vi "adjust.vi"(8 "error in (no error)":errorcluster, 11 "DL090216RangeOffsetImageProcessor in":refnum<class "ImageProcessorDL090216RangeOffset.lvclass">) -> (0 "error out":errorcluster, 3 "DL090216RangeOffsetImageProcessor out":refnum<class "ImageProcessorDL090216RangeOffset.lvclass">)   [LabVIEW 2010, in "ImageProcessorDL090216RangeOffset.lvclass"]
uses:
  ImageProcessorDL090216RangeOffset.lvclass
  common/clusters/range_offset_cluster.ctl
  ImageProcessorDL090216RangeOffset.lvclass/ImageProcessorDL090216RangeOffset.ctl
  GenericImageProcessor/GenericImageProcessor/GenericImageProcessor.lvclass
  Command/GenericImageProcessorChangedCommand/GenericImageProcessorChangedCommand/GenericImageProcessorChangedCommand.lvclass
panel:
  in  "done":bool
  in  "channels":T1[](array[typedef]) {"offset" min=0.0 max=1.0 step=0.0010000000474974513 scale=0.0..1.0; "range" min=0.0 max=1.0 step=0.0010000000474974513 scale=0.0..1.0}
  in  "optimise":bool
  in  "master":T1={"range"=7.119999645510688e-05, "offset"=0.10570889711380005} {"offset" min=0.0 max=1.0 step=0.0010000000474974513 scale=0.0..1.0; "range" min=0.0 max=1.0 step=0.0010000000474974513 scale=0.0..1.0}
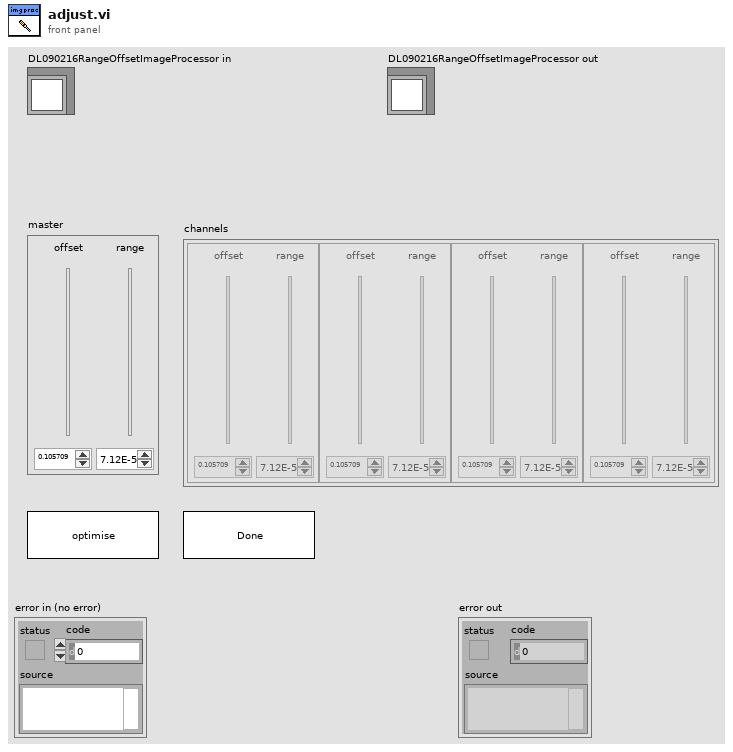
[diagram p1: front panel]
types:
  T1 = typedef "range_offset_cluster.ctl" = cluster{"range":dbl, "offset":dbl}
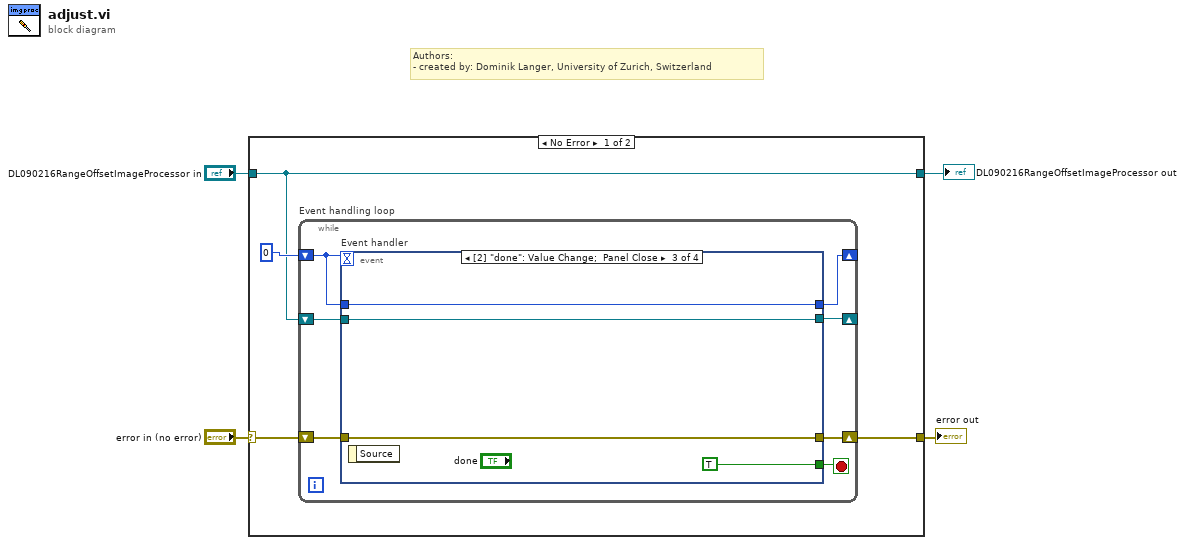
[diagram p0: block diagram]
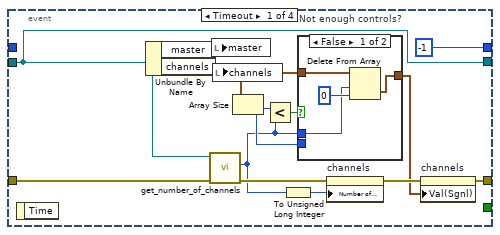
[diagram p2: hidden frame]
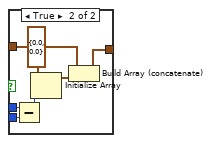
[diagram p3: hidden frame]
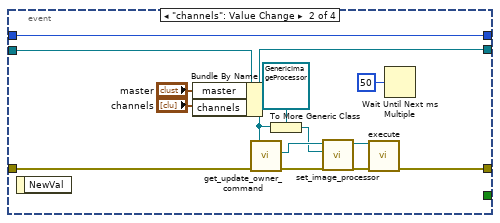
[diagram p4: hidden frame]
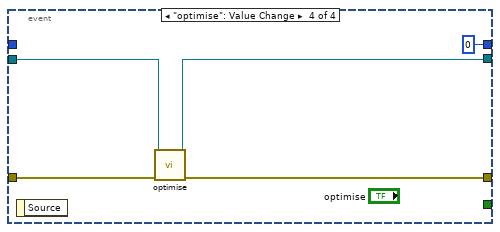
[diagram p5: hidden frame]
diagram:
  # "Authors: \n- created by: Dominik Langer, University of Zurich, Switzerland"
  n1 = case shown="No Error" "error in (no error)" {
    selector: "error in (no error)" -> [w8 w64]
    tunnel: [w7 w64] -> w3
    tunnel: [w5 w63] -> w2
    tunnel: "DL090216RangeOffsetImageProcessor in" -> [w5 w63]
    frame No Error {
      n2 = while "Event handling loop" {
        shift-right: [w14] -> w7
        shift-left: w8 -> [w15]
        shift-right: [w11] -> _
        shift-left: 0 -> [w12]
        shift-right: [w9] -> _
        shift-left: w5 -> [w10]
        stop <- w13 stop-if-true
        n3 = event "Event handler" shown="[2] \"done\": Value Change;  Panel Close" {
          selector: _ -> [_ _ _ _]
          dyn-events: _ -> [_ _ _ _]
          timeout: w12 -> [_ _ _ _]
          tunnel: w15 -> [w17 w49 w57 w59]
          tunnel: [w19 w51 w57 w58] -> w14
          tunnel: [_ _ TRUE _] -> w13
          tunnel: [-1 w53 w55 0] -> w11
          tunnel: w12 -> [_ w53 w55 _]
          tunnel: w10 -> [w16 w50 w54 w61]
          tunnel: [w16 w41 w54 w60] -> w9
          event Timeout {
            n4 = event-data() -> ()  [unwired: 2 out]
            n5 = Unbundle By Name(w16) -> ("master"=w28:T1, "channels"=w24:T1[])
            n6 = call "get_number_of_channels.vi"("error in (no error)"=w17, "GenericImageProcessor.lvclass in"=w16) -> ("error out"=w27:errorcluster, "number of channels"=w22:i32)  [unwired: 8 out]
            n7 = local write "master"(w28) -> ()
            n8 = local write "channels"(w24) -> ()
            n9 = Array Size(array=w24) -> (size(s)=w23:i32)
            n10 = Less?(x=w23, y=w22) -> (x < y?=w21:bool)
            n11 = To Unsigned Long Integer(number=w22) -> (unsigned 32bit integer=w26:u32)
            n12 = case "Not enough controls?" shown="False" w21 {
              tunnel: w22 -> [w30 w39]
              tunnel: w23 -> [_ w38]
              tunnel: w24 -> [w32 w35]
              tunnel: [w29 w33] -> w18
              frame False {
                n13 = Delete From Array(array=w32, length=w30, index=0) -> (deleted portion=w29:T1[])  [unwired: 1 out]
              }
              frame True {
                n14 = Subtract(x=w39, y=w38) -> (x-y=w37:i32)
                n15 = Initialize Array(T1 {"range"=0.0, "offset"=0.0} ("master"), w37) -> (w34:T1[])
                n16 = Build Array (concatenate)(w35, w34) -> (w33:T1[])
              }
            }
            n17 = property on="channels" class="Arr (strict)"(error in=w27, "Number of Columns"=w26) -> (error out=w20:errorcluster)  [unwired: 1 in, 1 out]
            n18 = property on="channels" class="Arr (strict)"(error in=w20, "Val(Sgnl)"=w18) -> (error out=w19:errorcluster)  [unwired: 1 in, 1 out]
          }
          event "channels": Value Change {
            n19 = event-data() -> ()  [unwired: 2 out]
            n20 = Bundle By Name(cluster=w50, "master"="master", "channels"="channels") -> (w41:refnum<class "ImageProcessorDL090216RangeOffset.lvclass">)
            n21 = call-dynamic "get_update_owner_command.vi"("error in (no error)"=w49, "GenericImageProcessor.lvclass in"=w41) -> ("error out"=w45:errorcluster, "update-owner command"=w47:refnum<class "GenericImageProcessorChangedCommand.lvclass">)  [unwired: 8 out]
            n22 = To More Generic Class(target class=refnum<class "GenericImageProcessor.lvclass"> refnum ("GenericImageProcessor.lvclass"), reference=w41) -> (generic class reference=w42:refnum<class "GenericImageProcessor.lvclass">)
            n23 = call-dynamic "set_image_processor.vi"("error in (no error)"=w45, "image processor"=w42, "GenericImageProcessorChangedCommand.lvclass in"=w47) -> ("error out"=w48:errorcluster, "GenericImageProcessorChangedCommand.lvclass out"=w44:refnum<class "GenericImageProcessorChangedCommand.lvclass">)  [unwired: 7 out]
            n24 = call-dynamic "execute.vi"("error in (no error)"=w48, "GenericCommand in"=w44) -> ("error out"=w51:errorcluster)  [unwired: 9 out]
            n25 = Wait Until Next ms Multiple(millisecond multiple=u32 50) -> ()  [unwired: 1 out]
          }
          event "done": Value Change; Panel Close {
            n26 = event-data() -> ()  [unwired: 2 out]
          }
          event "optimise": Value Change {
            n27 = event-data() -> ()  [unwired: 2 out]
            n28 = call-dynamic "optimise.vi"("error in (no error)"=w59, "DL090216RangeOffsetImageProcessor in"=w61) -> ("error out"=w58:errorcluster, "DL090216RangeOffsetImageProcessor out"=w60:refnum<class "ImageProcessorDL090216RangeOffset.lvclass">)  [unwired: 8 out]
          }
        }
      }
    }
    frame Error {
    }
  }
  "error out" <- w3
  "DL090216RangeOffsetImageProcessor out" <- w2
